vi "VSI Read Bits.vi"(6 "ReadBitsNum":i32, 7 "pReadBitStr":string, 9 "SPIIndex":i32, 10 "DevIndex":i32, 11 "DevType":i32) -> (3 "function return":i32, 5 "pReadBitStr out":string)   [LabVIEW 2010, in "ControlSPI.lvlib"]
doc: "int WINAPI VSI_ReadBits(int DevType,int DevIndex,int SPIIndex,unsigned char *pReadBitStr,int ReadBitsNum);"
uses:
  ControlSPI.lvlib
  ControlSPI/Ginkgo_Driver.dll
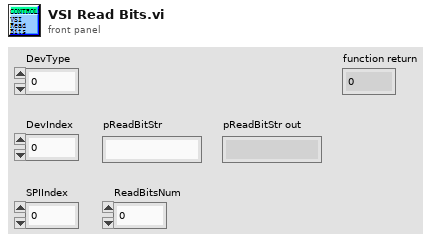
[diagram p1: front panel]
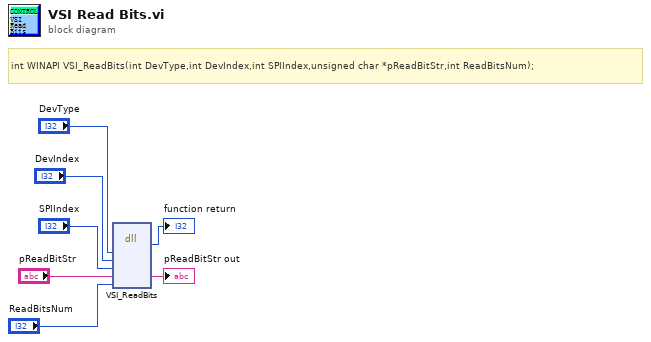
[diagram p0: block diagram]
diagram:
  # "int WINAPI VSI_ReadBits(int DevType,int DevIndex,int SPIIndex,unsigned char *pReadBitStr,int ReadBitsNum);"
  n1 = dll-call lib="E:/Project/vt_ginkgo/truck/Ginkgo Driver/vs2010/Ginkgo_USB-I2C&SPI&CAN_API_v2.0.3.3/lib/labview_32bit/ControlSPI/Ginkgo_Driver.*" fn="VSI_ReadBits"("DevType"="DevType", "DevIndex"="DevIndex", "SPIIndex"="SPIIndex", "pReadBitStr"="pReadBitStr", "ReadBitsNum"="ReadBitsNum") -> (→"function return":i32, "pReadBitStr"=→"pReadBitStr out":string)  [unwired: 7 in, 2 out]
